vi "transmitMessageEvent.vi"(4 "MessageEvent":refnum<user-event>, 5 "Event Data":T1, 6 "Control Ref":refnum<k24>, 7 "Event Common Data":T2) -> ()   [LabVIEW 2013, in "SLMControl.lvlib" / "SM1000.lvclass"]
doc: "Handles any received 'OnConnect'-events from an EC device session.\nEvnets are only detected after registration through the 'registerConnectEvent' method."
uses:
  SM1000.lvclass
  C:/Users/vangeste/Desktop/2015-06-02 - SLM - MAIF/HC-HardwareCharacterization/Sources/SM1000/LECSession.dll
  HC-HardwareCharacterization/Sources/SM1000/LECSession.dll
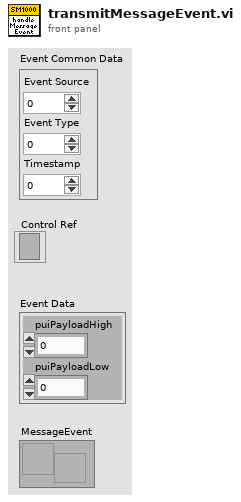
[diagram p1: front panel]
types:
  T1 = cluster{"puiPayloadHigh":u32, "puiPayloadLow":u32}
  T2 = cluster{"Event Source":i32, "Event Type":u32, "Timestamp":u32}
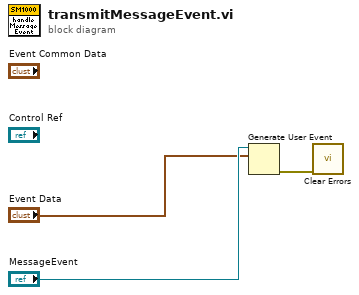
[diagram p0: block diagram]
diagram:
  n1 = Generate User Event(user event="MessageEvent", event data cluster="Event Data") -> (error out=w3:errorcluster)  [unwired: 2 in, 1 out]
  n2 = call <vilib>:"Clear Errors.vi"("error in (no error)"=w3) -> ()  [unwired: 6 in, 1 out]
